vi "INIT.vi"(8 "error in (no error)":errorcluster, 11 "UV-VIS-Avantes in":refnum<class "UV-VIS-Avantes.lvclass">) -> (0 "error out":errorcluster, 3 "UV-VIS-Avantes out":refnum<class "UV-VIS-Avantes.lvclass">)   [LabVIEW 2015, in "UV-VIS-Avantes.lvclass"]
uses:
  UV-VIS-Avantes.lvclass
  Detector.lvclass
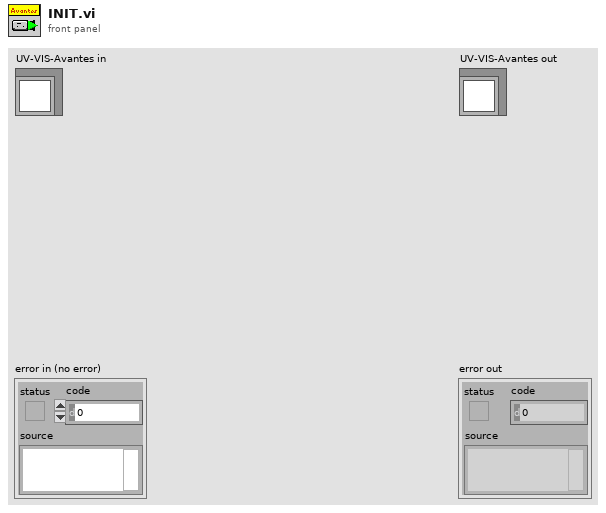
[diagram p1: front panel]
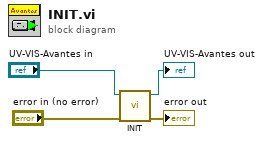
[diagram p0: block diagram]
diagram:
  n1 = call-parent "INIT.vi"("error in (no error)"="error in (no error)", "GeneralFunctionality in"="UV-VIS-Avantes in") -> ("error out"=→"error out":errorcluster, "GeneralFunctionality out"=→"UV-VIS-Avantes out":refnum<class "UV-VIS-Avantes.lvclass">)  [unwired: 8 in]
